vi "UnescapeURI.vi"(11 "Escaped URI":string) -> (3 "URI":string)   [LabVIEW 2017, in "URI.lvlib"]
doc: "Decodes the percent-encoded sequences in an escaped URI."
uses:
  URI.lvlib
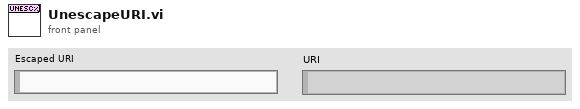
[diagram p1: front panel]
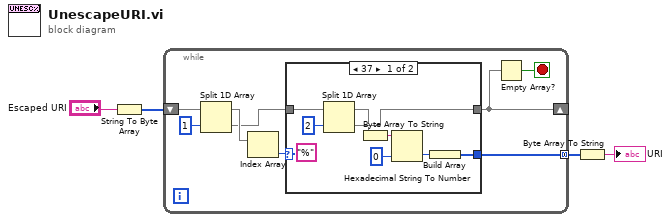
[diagram p0: block diagram]
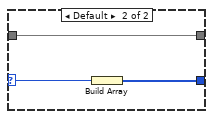
[diagram p2: hidden frame]
diagram:
  n1 = String To Byte Array(string="Escaped URI") -> (unsigned byte array=w2:u8[])
  n2 = while {
    shift-right: [w5] -> _
    shift-left: w2 -> [w12]
    tunnel: [w6] -> w1 mode=concatenating
    stop <- w9 stop-if-true
    n3 = Split 1D Array(array=w12, index=1) -> (first subarray=w10:u8[], second subarray=w7:u8[])
    n4 = Index Array(array=w10) -> (element=w8:u8)  [unwired: 1 in]
    n5 = case shown="37" w8 {
      selector: w8 -> [_ w22]
      tunnel: w7 -> [w19 w23]
      tunnel: [w18 w23] -> w5
      tunnel: [w14 w21] -> w6
      frame 37 {
        (unwired) "%" ("regular expression")
        n6 = Split 1D Array(array=w19, index=2) -> (first subarray=w17:u8[], second subarray=w18:u8[])
        n7 = Byte Array To String(unsigned byte array=w17) -> (string=w16:string)
        n8 = Hexadecimal String To Number(string=w16, default (0uL)=u8 0 ("default (0 U32)")) -> (number=w15:u8)  [unwired: 1 in, 1 out]
        n9 = Build Array(w15) -> (w14:u8[])
      }
      frame Default {
        n10 = Build Array(w22) -> (w21:u8[])
      }
    }
    n11 = Empty Array?(array=w5) -> (empty?=w9:bool)
  }
  n12 = Byte Array To String(unsigned byte array=w1) -> (string=→"URI":string)
